vi "CS POLARIS BME DG Client.i attribute.vi"(0 "VI Refnum":refnum<vi>, 2 "CLASS.i attribute":T1, 3 "Action":T2(ring), 5 "error in (no error)":errorcluster) -> (14 "VI Refnum out":refnum<vi>, 16 "CLASS.i attribute out":T1, 19 "error out":errorcluster)   [LabVIEW 2009, in "CS POLARIS BME DG Client.lvlib"]
doc: "This is a so-called functional global variable. It manages the access to a global variable in a thread-safe way. \n\nHere the attribute data of all instances of THIS class are stored. This is done for performance reasons.\n\nLicense Agreement for this software:\n\nCopyright (C)\nGesellschaft für Schwerionenforschung, GSI\nPlanckstr. 1\n64291 Darmstadt\nGermany\n\nContact: D.Beck@gsi.de \n\nThis program is free software; you can redistribute it and/or modify it under the terms of the GNU General Public License as published by the Free Software Foundation; either version 2 of the license, or (at your option) any later version.\n\nThis program is distributed in the hope that it will be useful, but WITHOUT ANY WARRANTY; without even the implied warranty of MERCHANTABILITY or FITNESS FOR A PARTICULAR PURPOSE. See the GNU General License for more details (http://www.gnu.org).\n\nGesellschaft für Schwerionenforschung, GSI\nPlanckstr. 1, 64291 Darmstadt, Germany\nFor all questions and ideas contact: M.Richter@gsi.de, H.Brand@gsi.de or D.Beck@gsi.de.\nLast update: 17-JUN-2004"
uses:
  CS POLARIS BME DG Client.lvlib
  CS POLARIS BME DG Client.i attribute.ctl
  CSCore/CSSystem/CoreDefs/CoreDefs.error_type.ctl
  CSCore/CSSystem/CoreLib/CoreLib.lvlib
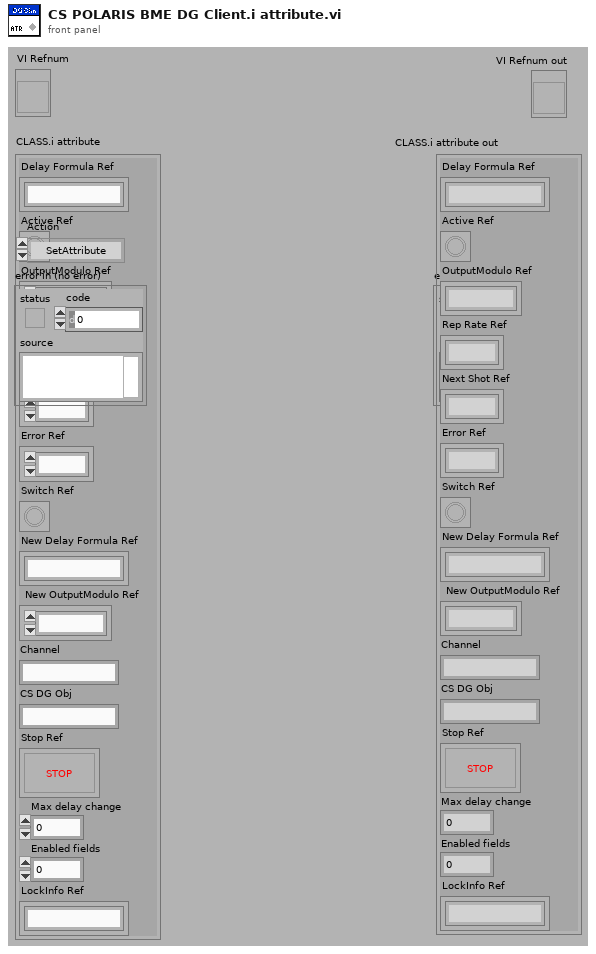
[diagram p1: front panel]
types:
  T1 = typedef "CS POLARIS BME DG Client.lvlib/CS POLARIS BME DG Client.i attribute.ctl" = cluster{"Delay Formula Ref":refnum<vi>, "Active Ref":refnum<vi>, "OutputModulo Ref":refnum<vi>, "Rep Rate Ref":refnum<vi>, "Next Shot Ref":refnum<vi>, "Error Ref":refnum<vi>, "Switch Ref":refnum<vi>, "New Delay Formula Ref":refnum<vi>, "New OutputModulo Ref ":refnum<vi>, "Channel":string, "CS DG Obj":string, "Stop Ref":refnum<vi>, "Max delay change":dbl, "Enabled fields":u8, "LockInfo Ref":refnum<vi>}
  T2 = enum16{"SetAttribute", "GetAttribute", "CreateAttribute", "DestroyAttribute", "DestroyAllAtributes"}
  T3 = typedef "CoreDefs.error_type.ctl" = enum16{"no error", "can't load process", "can't unload process", "process does not exist", "can't install process", "can't remove process", "unknown function", "time out", "can't execute function", "duplicate queue name", "super not found", "caller queue invalid", "can't ping process", "unknown error", "VISA Error", "VISA timeout", "GPIB timeout", "GPIB error", "communication error", "data type mismatch", "can't read data from OPC server", "can't write data to OPC server", "OET error", "function not implemented", "process already exists", "invalid Shared Variable name", "error writing Shared Variable", "error reading Shared Variable", "invalid client name", "corrupt database", "unknown class", "call not authorized", "parameter out of range", "OET timeout: can't get data to modify", "invalid queue name", "requested operation incompatible with current state", "event undefined", "event disabled", "state undefined", "caller is not a friend", "EventBuilder: bad eventID", "EventBuilder: no DAQ devices", "a thread must not stop itself", "UNUSED ELEMENT4", "DiscArchiver: eventData incomplete", "DiscArchiver: eventData does not belong to run", "DiscArchiver: can't open file", "DiscArchiver: can't write to file", "DiscArchiver: available disc space low", "can't acquire semaphore", "error reading data from database", "notifier object is not existing", "can't register process", "can't unregister process", "illegal event type", "object disabled", "object already exists", "can't change state", "Instrument not found", "no connection to remote node", "invalid reference", "N/A", "UNUSED ELEMENT 1", "element not found", "illegal TCP/IP connection detected", "object does not exist", "invalid access ID", "unknown CS system", "invalid privilige", "unsupported data type", "unsupported server type", "IO server already exists", "Shared Variable already exists"}
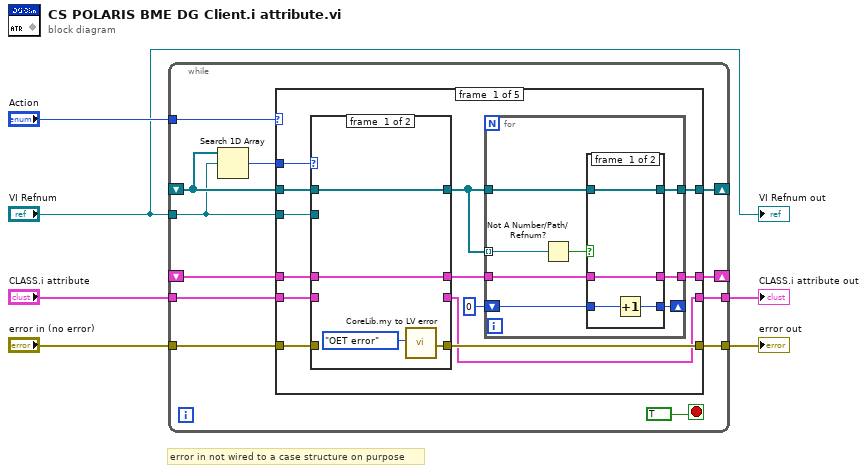
[diagram p0: block diagram]
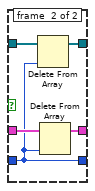
[diagram p2: hidden frame]
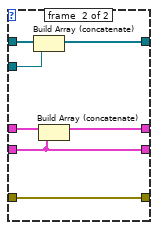
[diagram p3: hidden frame]
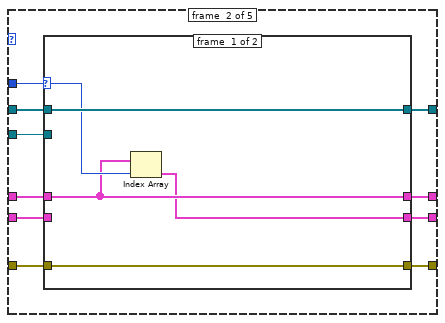
[diagram p4: hidden frame]
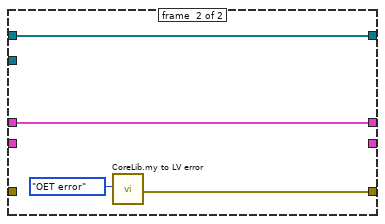
[diagram p5: hidden frame]
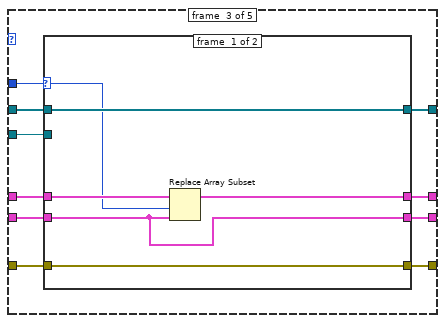
[diagram p6: hidden frame]
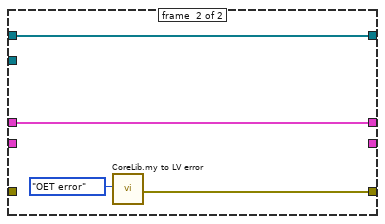
[diagram p7: hidden frame]
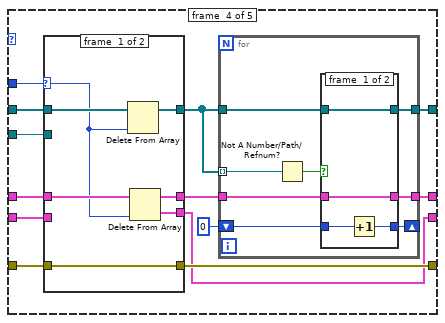
[diagram p8: hidden frame]
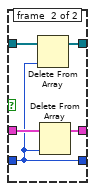
[diagram p9: hidden frame]
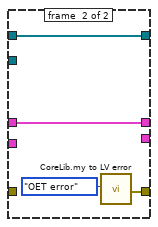
[diagram p10: hidden frame]
diagram:
  # "error in not wired to a case structure on purpose"
  n1 = while {
    shift-right: [w12] -> _
    shift-left: _ -> [w13]
    tunnel: "Action" -> [w17]
    shift-right: [w14] -> _
    shift-left: _ -> [w10]
    tunnel: "VI Refnum" -> [w9]
    tunnel: "error in (no error)" -> [w16]
    tunnel: [w15] -> w4
    tunnel: "CLASS.i attribute" -> [w11]
    tunnel: [w7] -> w1
    stop <- TRUE stop-if-true
    n2 = Search 1D Array(1D array=w10, element=w9) -> (index of element=w8:i32)  [unwired: 1 in]
    n3 = case shown="\"CreateAttribute\"" w17 {
      tunnel: w10 -> [w29 w67 w86 w109 _]
      tunnel: w9 -> [w28 w65 w84 w108 _]
      tunnel: w16 -> [w31 w69 w88 w111 w140]
      tunnel: [w30 w68 w87 w110 w140] -> w15
      tunnel: [w23 w66 w85 w103 _] -> w14
      tunnel: w13 -> [w27 w64 w83 w107 _]
      tunnel: [w22 w63 w82 w101 _] -> w12
      tunnel: w11 -> [w26 w62 w81 w106 _]
      tunnel: w8 -> [w25 w61 w80 w105 _]
      tunnel: [w19 w60 w79 w99 _] -> w7
      frame #0 {
        n4 = case shown="-1" w25 {
          tunnel: w31 -> [_ w59]
          tunnel: [w51 w59] -> w30
          tunnel: w29 -> [w50 w58]
          tunnel: [w50 w57] -> w21
          tunnel: w28 -> [_ w56]
          tunnel: w27 -> [w49 w55]
          tunnel: [w49 w54] -> w20
          tunnel: w26 -> [_ w53]
          tunnel: [_ w53] -> w19
          frame #0 {
            n5 = call "CoreLib.my to LV error.vi"("ErrorTypes"=CoreDefs.error_type."OET error") -> ("myErrorCluster"=w51:errorcluster)  [unwired: 17 in, 1 out]
          }
          frame #1 {
            n6 = Build Array (concatenate)(w58, w56) -> (w57:refnum<vi>[])
            n7 = Build Array (concatenate)(w55, w53) -> (w54:T1[])
          }
        }
        n8 = for {
          tunnel: w21 -> [w36]
          tunnel: [w35] -> w23
          tunnel: [w39] -> w22
          tunnel: w20 -> [w38]
          tunnel: w21 -> [w34] mode=indexing
          shift-right: [w33] -> _
          shift-left: 0 -> [w32]
          n9 = Not A Number/Path/Refnum?(number/path/refnum=w34) -> (NaN/Path/Refnum?=w37:bool)
          n10 = case shown="True" w37 {
            tunnel: [w43 w48] -> w39
            tunnel: w38 -> [w43 w47]
            tunnel: [w42 w45] -> w35
            tunnel: w36 -> [w42 w46]
            tunnel: w32 -> [w41 w44]
            tunnel: [w40 w44] -> w33
            frame #0 {
              n11 = Increment(x=w41) -> (x+1=w40:i32)
            }
            frame #1 {
              n12 = Delete From Array(array=w46, index=w44) -> (array with subset deleted=w45:refnum<vi>[])  [unwired: 1 in, 1 out]
              n13 = Delete From Array(array=w47, index=w44) -> (array with subset deleted=w48:T1[])  [unwired: 1 in, 1 out]
            }
          }
        }
      }
      frame #1 {
        n14 = case shown="0, Default" w61 {
          selector: w61 -> [w72 _]
          tunnel: w69 -> [w74 _]
          tunnel: [w74 w77] -> w68
          tunnel: w67 -> [w73 w76]
          tunnel: [w73 w76] -> w66
          tunnel: w65 -> [_ _]
          tunnel: w64 -> [w71 w75]
          tunnel: [w71 w75] -> w63
          tunnel: w62 -> [_ _]
          tunnel: [w70 _] -> w60
          frame #0 {
            n15 = Index Array(array=w71, index=w72) -> (element=w70:T1)
          }
          frame #1 {
            n16 = call "CoreLib.my to LV error.vi"("ErrorTypes"=CoreDefs.error_type."OET error") -> ("myErrorCluster"=w77:errorcluster)  [unwired: 17 in, 1 out]
          }
        }
      }
      frame #2 {
        n17 = case shown="0, Default" w80 {
          selector: w80 -> [w90 _]
          tunnel: w88 -> [w94 _]
          tunnel: [w94 w97] -> w87
          tunnel: w86 -> [w93 w96]
          tunnel: [w93 w96] -> w85
          tunnel: w84 -> [_ _]
          tunnel: w83 -> [w92 w95]
          tunnel: [w91 w95] -> w82
          tunnel: w81 -> [w89 _]
          tunnel: [w89 _] -> w79
          frame #0 {
            n18 = Replace Array Subset(array=w92, new element=w89, index=w90) -> (w91:T1[])
          }
          frame #1 {
            n19 = call "CoreLib.my to LV error.vi"("ErrorTypes"=CoreDefs.error_type."OET error") -> ("myErrorCluster"=w97:errorcluster)  [unwired: 17 in, 1 out]
          }
        }
      }
      frame #3 {
        n20 = case shown="-1" w105 {
          selector: w105 -> [w131 _]
          tunnel: w111 -> [w135 _]
          tunnel: [w135 w138] -> w110
          tunnel: w109 -> [w134 w137]
          tunnel: [w133 w137] -> w102
          tunnel: w108 -> [_ _]
          tunnel: w107 -> [w132 w136]
          tunnel: [w130 w136] -> w100
          tunnel: w106 -> [_ _]
          tunnel: [w129 _] -> w99
          frame #0 {
            n21 = Delete From Array(array=w134, index=w131) -> (array with subset deleted=w133:refnum<vi>[])  [unwired: 1 in, 1 out]
            n22 = Delete From Array(array=w132, index=w131) -> (deleted portion=w129:T1, array with subset deleted=w130:T1[])  [unwired: 1 in]
          }
          frame #1 {
            n23 = call "CoreLib.my to LV error.vi"("ErrorTypes"=CoreDefs.error_type."OET error") -> ("myErrorCluster"=w138:errorcluster)  [unwired: 17 in, 1 out]
          }
        }
        n24 = for {
          tunnel: w102 -> [w116]
          tunnel: [w115] -> w103
          tunnel: [w119] -> w101
          tunnel: w100 -> [w118]
          tunnel: w102 -> [w114] mode=indexing
          shift-right: [w113] -> _
          shift-left: 0 -> [w112]
          n25 = Not A Number/Path/Refnum?(number/path/refnum=w114) -> (NaN/Path/Refnum?=w117:bool)
          n26 = case shown="True" w117 {
            tunnel: [w123 w128] -> w119
            tunnel: w118 -> [w123 w127]
            tunnel: [w122 w125] -> w115
            tunnel: w116 -> [w122 w126]
            tunnel: w112 -> [w121 w124]
            tunnel: [w120 w124] -> w113
            frame #0 {
              n27 = Increment(x=w121) -> (x+1=w120:i32)
            }
            frame #1 {
              n28 = Delete From Array(array=w126, index=w124) -> (array with subset deleted=w125:refnum<vi>[])  [unwired: 1 in, 1 out]
              n29 = Delete From Array(array=w127, index=w124) -> (array with subset deleted=w128:T1[])  [unwired: 1 in, 1 out]
            }
          }
        }
      }
      frame #4 {
      }
    }
  }
  "error out" <- w4
  "CLASS.i attribute out" <- w1
  "VI Refnum out" <- "VI Refnum"
